vi "network stream read.vi"(8 "error in (no error)":errorcluster, 11 "endpoint in":refnum<k21>) -> (0 "error out":errorcluster, 2 "Data":fxp<+/-,17,5> format="%#_17g", 3 "endpoint out":refnum<k21>)   [LabVIEW 2024]
uses:
  <resource>/objmgr/ni.dex.rc
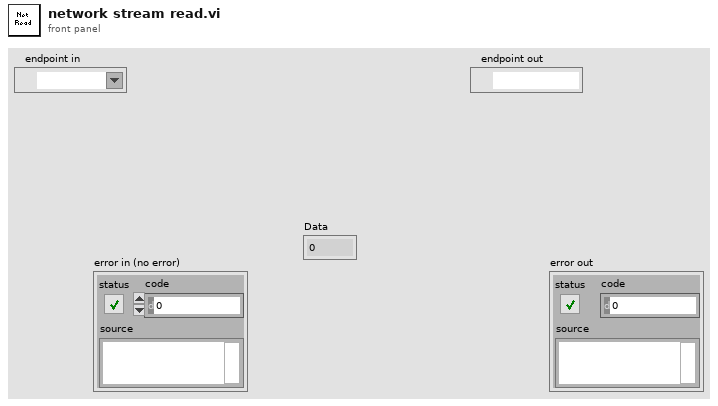
[diagram p1: front panel]
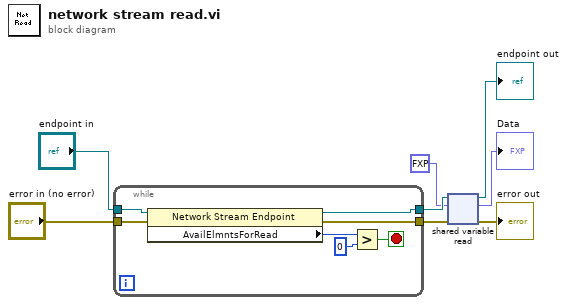
[diagram p0: block diagram]
diagram:
  n1 = while {
    tunnel: "error in (no error)" -> [w15]
    tunnel: [w11] -> w7
    tunnel: [w10] -> w4
    tunnel: "endpoint in" -> [w9]
    stop <- w12 stop-if-true
    n2 = property class="Network Stream Endpoint"(reference=w9, error in=w15) -> (reference out=w10:refnum<k21>, error out=w11:errorcluster, "AvailElmntsForRead"=w14:i32)
    n3 = Greater?(x=w14, y=0) -> (0:w12:bool)
  }
  n4 = shared-variable-read(w4, w7, fxp<+/-,17,5> 0.0 ("data type")) -> (→"endpoint out":refnum<k21>, →"error out":errorcluster, →"Data":fxp<+/-,17,5>)  [unwired: 1 in, 1 out]
